vi "Main.vi"(11 "Module Admin":refnum<class "Delacor_lib_QMH_Module Admin.lvclass">) -> ()   [LabVIEW 2022 SP3, in "UI Manager.lvlib"]
doc: "The UI Manager module forms the visual framework that other modules are displayed in. It contains the basic user interface of the application (menu bar, header, content area, footer).\n____\nHAMPEL SOFTWARE ENGINEERING v2.6.0 (2023-12-19 10:54)"
uses:
  UI Manager.lvlib
  <vilib>/Delacor/Delacor QMH/Libraries/Module Admin_class/Delacor_lib_QMH_Module Admin.lvclass
  Libraries/hse-libraries/Source/hse-dqmh/Controls/System Message Argument--cluster.ctl
  Libraries/hse-libraries/Source/hse-dqmh/Controls/System Message Source.ctl
  Module Data--cluster.ctl
  Libraries/hse-libraries/Source/hse-configuration/config-base/config-base.lvclass
  SubVIs/Layout References--cluster.ctl
  SubVIs/SubPanels--map.ctl
  SubVIs/SubPnl Map References--cluster.ctl
  Login Argument--cluster.ctl
  <vilib>/Delacor/Delacor QMH/Libraries/Message Queue_class/Delacor_lib_QMH_Message Queue.lvclass/Delacor_lib_QMH_Message Queue.ctl
  Stop Argument--cluster.ctl
  Shutdown Application Argument--cluster.ctl
  Add Module to Run-Time Menu Argument--cluster.ctl
  Libraries/hse-libraries/Source/hse-dqmh/Controls/System Message - Add to Run-Time Menu - Argument--cluster.ctl
  Remove Module from Run-Time Menu Argument--cluster.ctl
  Libraries/hse-libraries/Source/hse-dqmh/Controls/System Message - Remove from Run-Time Menu - Argument--cluster.ctl
  Load Module Into Subpanel Argument--cluster.ctl
  Libraries/hse-libraries/Source/hse-dqmh/Controls/System Message - Ready for Display - Payload--cluster.ctl
  Configure Argument--cluster.ctl
  Prepare Argument--cluster.ctl
  Set Modules Argument--cluster.ctl
  Set Modules (Reply Payload)--cluster.ctl
  Set Run-Time Menu Argument--cluster.ctl
  Show HSE-ABOUT Argument--cluster.ctl
  Show PROJECT-ABOUT Argument--cluster.ctl
  Update Status Bar Argument--cluster.ctl
  Trigger System Message Argument--cluster.ctl
  Display another Module UI Argument--cluster.ctl
  Module Display Scenarios.ctl
  Set Run-Time Menu Visibility Argument--cluster.ctl
  Set Window Closeable State Argument--cluster.ctl
  Set CLI Arguments Argument--cluster.ctl
  Set CLI Arguments (Reply Payload)--cluster.ctl
  Get CLI Arguments Argument--cluster.ctl
  Get CLI Arguments (Reply Payload)--cluster.ctl
  External Login Argument--cluster.ctl
  Get User Level Argument--cluster.ctl
  Get User Level (Reply Payload)--cluster.ctl
  <vilib>/Delacor/Delacor QMH/Libraries/Module Admin_class/Delacor_lib_QMH_Module Admin.lvclass/Delacor_lib_QMH_Module Admin.ctl
  Libraries/hse-libraries/Source/hse-application/hse-application.lvclass/hse-application.ctl
  <vilib>/Delacor/Delacor QMH/Libraries/Message Queue_class/Delacor_lib_QMH_Enqueue Message (Single).vi
  <vilib>/Delacor/Delacor QMH/Libraries/Module Admin_class/Delacor_lib_QMH_Get External Launch.vi
  Libraries/hse-libraries/Source/hse-application/HSE Application not initialized--error.vi
  Libraries/hse-libraries/Source/hse-configuration/config-ini/config-ini.lvclass
  C:/Projects/579-Intelligent-Systems-Term-Project/06_Source/UI/FReVSys_Source/Libraries/hse-libraries/Source/hse-configuration/config-base/config-base.lvclass
  Libraries/hse-libraries/Source/hse-application/hse-application__GetSingleton.vi
  <vilib>/Utility/error.llb/Error Cluster From Error Code.vi
  Project/PROJECT_Evaluate Default Menu Selection.vi
  Project/PROJECT_UserCredentials.vi
  <vilib>/ErrorRing/Error Ring.xnode
  <vilib>/Delacor/Delacor QMH/Libraries/Message Queue_class/Delacor_lib_QMH_Message Queue.lvclass
  Libraries/hse-libraries/Source/hse-ui/hse-ui.lvlib
  Libraries/hse-libraries/Source/hse-application/hse-application.lvclass
  Libraries/hse-libraries/Source/hse-dqmh/hse-dqmh.lvlib
  <vilib>/Hampel Software Engineering/HSE Logger/hse-logger.lvlib
  Project/Project.lvlib
panel:
  out "Status Bar":string
  out "error out":errorcluster
  out "Version":string
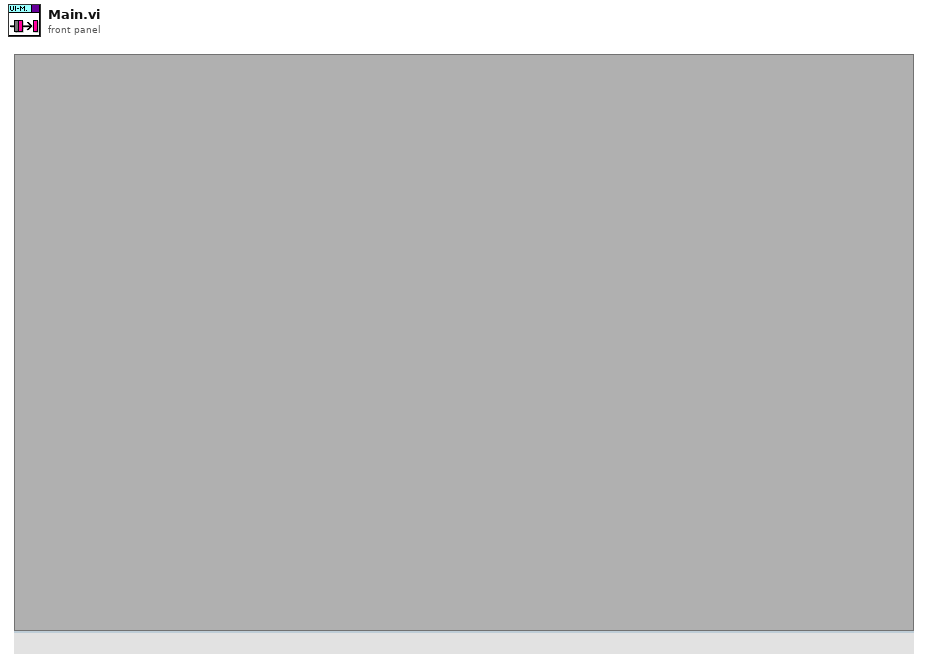
[diagram p1: front panel]
types:
  T1 = typedef "UI Manager.lvlib/Request Events--cluster.ctl" = cluster{"Stop Module":refnum<user-event>, "Show Panel":refnum<user-event>, "Hide Panel":refnum<user-event>, "Get Module Execution Status":refnum<user-event>, "Show Diagram":refnum<user-event>, "Set Run-Time Menu":refnum<user-event>, "Show HSE-ABOUT":refnum<user-event>, "Show PROJECT-ABOUT":refnum<user-event>, "Configure":refnum<user-event>, "Prepare":refnum<user-event>, "Update Status Bar":refnum<user-event>, "Trigger System Message":refnum<user-event>, "Add Module to Run-Time Menu":refnum<user-event>, "Set Modules":refnum<user-event>, "Register for Module Events":refnum<user-event>, "Display another Module UI":refnum<user-event>, "Set Run-Time Menu Visibility":refnum<user-event>, "Set Window Closeable State":refnum<user-event>, "Shutdown Application":refnum<user-event>, "Remove Module from Run-Time Menu":refnum<user-event>, "Set CLI Arguments":refnum<user-event>, "Get CLI Arguments":refnum<user-event>, "External Login":refnum<user-event>, "Get User Level":refnum<user-event>}
  T2 = typedef "UI Manager.lvlib/Module Data--cluster.ctl" = cluster{"hse-config":refnum<class "config-base.lvclass">, "Module Paths":path[], "Default Title":string, "Layout":T3, "CLI Arguments":string[], "Login Argument":T6}
  T3 = typedef "UI Manager.lvlib/Layout References--cluster.ctl" = cluster{"Layout-VI Ref":refnum<vi>, "SP_Content Ref":refnum<vi>, "Subpanel VI Ref":refnum<vi>, "STR_Headline":refnum<vi>, "SubPanels":T4}
  T4 = typedef "UI Manager.lvlib/SubPanels--map.ctl" = map{string, T5}
  T5 = typedef "UI Manager.lvlib/SubPnl Map References--cluster.ctl" = cluster{"SubPnl Refnum":refnum<vi>, "VI Refnum":refnum<vi>}
  T6 = typedef "UI Manager.lvlib/Login Argument--cluster.ctl" = cluster{"User Name":string, "User Level":string}
  T7 = enum32{"invalid lock state", "Not Locked", "Locked (No Password)", "Password-protected"}
  T8 = typedef "UI Manager.lvlib/Stop Argument--cluster.ctl" = cluster{"Origin":string, "Exit via Stop Module Req?":bool, "Wait for Module to stop?":bool}
  T9 = typedef "UI Manager.lvlib/Shutdown Application Argument--cluster.ctl" = cluster{"User Confirm?":bool}
  T10 = typedef "hse-dqmh.lvlib/System Message - Add to Run-Time Menu - Argument--cluster.ctl" = cluster{"Module Disk Path":path, "Module Descriptor":string}
  T11 = typedef "UI Manager.lvlib/Add Module to Run-Time Menu Argument--cluster.ctl" = cluster{"Module DQMH Path":path, "Module Descriptor":string}
  T12 = typedef "hse-dqmh.lvlib/System Message - Remove from Run-Time Menu - Argument--cluster.ctl" = cluster{"Module Disk Path":path}
  T13 = typedef "UI Manager.lvlib/Remove Module from Run-Time Menu Argument--cluster.ctl" = cluster{"Module DQMH Path":path}
  T14 = typedef "hse-dqmh.lvlib/System Message - Ready for Display - Payload--cluster.ctl" = cluster{"Module Path":path, "VI Reference":refnum<vi>, "Title":string, "Target SP Name":string}
  T15 = typedef "UI Manager.lvlib/Load Module Into Subpanel Argument--cluster.ctl" = cluster{"Module Path":path, "Module Name":string, "Title":string, "VI Reference":refnum<vi>, "Target SP Name":string}
  T16 = typedef "UI Manager.lvlib/Configure Argument--cluster.ctl" = cluster{"Boolean":bool}
  T17 = typedef "UI Manager.lvlib/Prepare Argument--cluster.ctl" = cluster{"Boolean":bool}
  T18 = typedef "UI Manager.lvlib/Set Modules Argument--cluster.ctl" = cluster{"Module Paths":path[], "Wait Notifier":refnum<notifier>, "wait for reply":bool}
  T19 = typedef "UI Manager.lvlib/Set Run-Time Menu Argument--cluster.ctl" = cluster{"Run-Time Menu Path":path}
  T20 = typedef "UI Manager.lvlib/Show HSE-ABOUT Argument--cluster.ctl" = cluster{"Boolean":bool}
  T21 = typedef "UI Manager.lvlib/Show PROJECT-ABOUT Argument--cluster.ctl" = cluster{"Boolean":bool}
  T22 = typedef "UI Manager.lvlib/Update Status Bar Argument--cluster.ctl" = cluster{"Status Message":string}
  T23 = typedef "UI Manager.lvlib/Trigger System Message Argument--cluster.ctl" = cluster{"Boolean":bool}
  T24 = typedef "UI Manager.lvlib/Display another Module UI Argument--cluster.ctl" = cluster{"Module DQMH Path":path, "Display Scenario":T25}
  T25 = typedef "UI Manager.lvlib/Module Display Scenarios.ctl" = enum16{"Stand-Alone", "Managed"}
  T26 = typedef "UI Manager.lvlib/Set Run-Time Menu Visibility Argument--cluster.ctl" = cluster{"Visible?":bool}
  T27 = typedef "UI Manager.lvlib/Set Window Closeable State Argument--cluster.ctl" = cluster{"Closeable?":bool}
  T28 = typedef "UI Manager.lvlib/Set CLI Arguments Argument--cluster.ctl" = cluster{"CLI Arguments":string[], "Wait Notifier":refnum<notifier>, "wait for reply":bool}
  T29 = typedef "UI Manager.lvlib/Get CLI Arguments Argument--cluster.ctl" = cluster{"Wait Notifier":refnum<notifier>, "wait for reply":bool}
  T30 = typedef "UI Manager.lvlib/External Login Argument--cluster.ctl" = cluster{"User Name":string, "User Level":string}
  T31 = typedef "UI Manager.lvlib/Get User Level Argument--cluster.ctl" = cluster{"Wait Notifier":refnum<notifier>, "wait for reply":bool}
  T32 = enum32{"Invalid", "Standard", "Closed", "Hidden", "Minimized", "Maximized"}
  T33 = typedef "UI Manager.lvlib/Set Modules (Reply Payload)--cluster.ctl" = cluster{"error":errorcluster}
  T34 = typedef "UI Manager.lvlib/Set CLI Arguments (Reply Payload)--cluster.ctl" = cluster{"error":errorcluster}
  T35 = typedef "UI Manager.lvlib/Get CLI Arguments (Reply Payload)--cluster.ctl" = cluster{"CLI Arguments":string[], "error":errorcluster}
  T36 = typedef "UI Manager.lvlib/Get User Level (Reply Payload)--cluster.ctl" = cluster{"User Name":string, "User Level":string, "error":errorcluster}
  T37 = typedef "eventvkey.ctl" = enum16{"ASCII", "Enter", "Return", "Shift", "Ctrl", "Alt", "Cmd", "Opt", "Caps", "NumLock", "Clear", "Break", "Up", "Down", "Left", "Right", "Insert", "Delete", "Home", "End", "PageUp", "PageDown", "Escape", "Help", "Pause", "ScrollLock", "F1", "F2", "F3", "F4", "F5", "F6", "F7", "F8", "F9", "F10", "F11", "F12", "F13", "F14", "F15", "F16", "F17", "F18", "F19", "F20", "F21", "F22", "F23", "F24", "Play", "VolumeUp", "VolumeDown", "Mute", "Two Byte Char"}
  T38 = cluster{"Shift":bool, "Ctrl":bool, "Alt":bool, "Cmd":bool, "Opt":bool}
  T39 = typedef "hse-dqmh.lvlib/System Message Source.ctl" = enum16{"module", "application", "network"}
  T40 = typedef "hse-dqmh.lvlib/Module Types.ctl" = enum16{"Singleton", "Cloneable"}
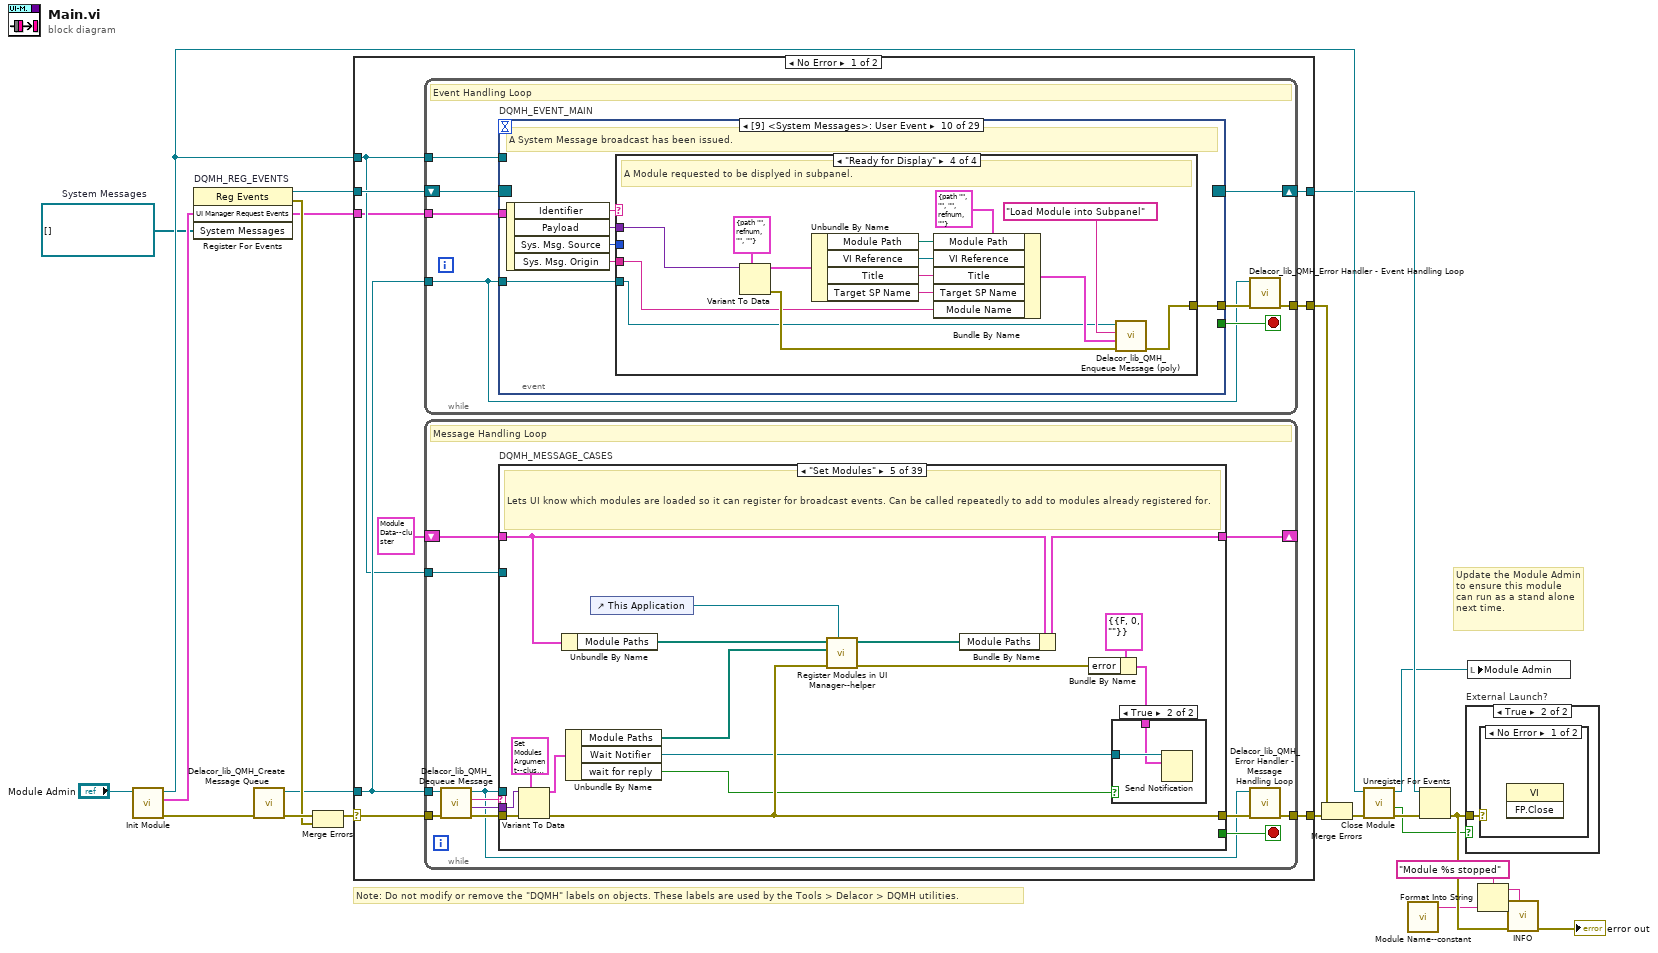
[diagram p0: block diagram]
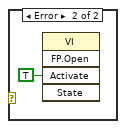
[diagram p3: hidden frame]
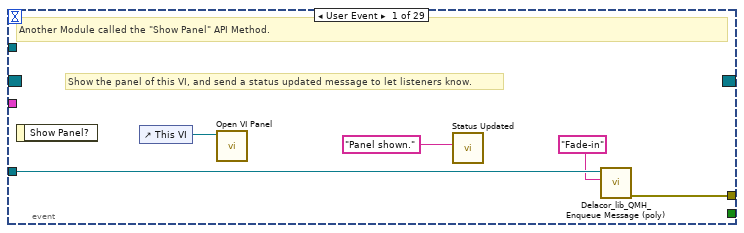
[diagram p4: hidden frame]
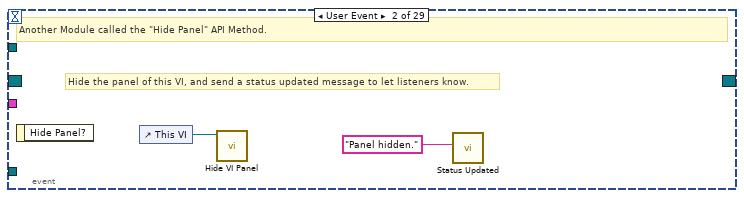
[diagram p5: hidden frame]
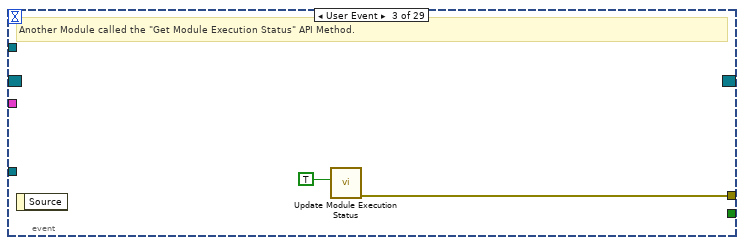
[diagram p6: hidden frame]
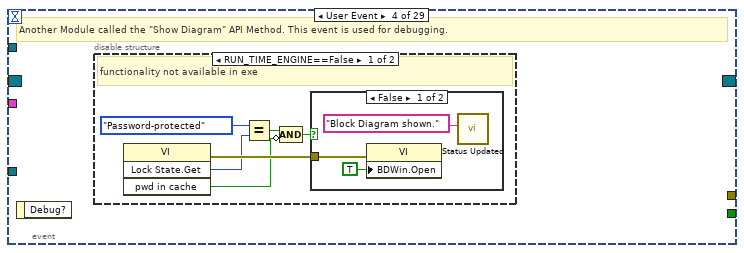
[diagram p7: hidden frame]
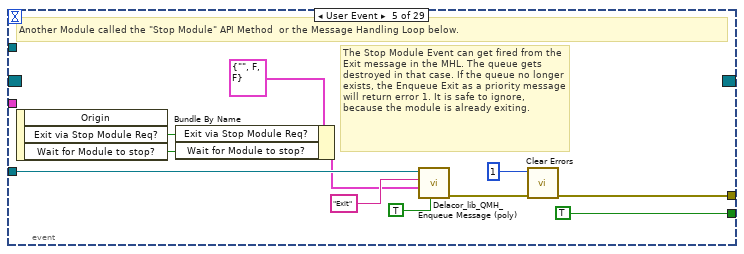
[diagram p10: hidden frame]
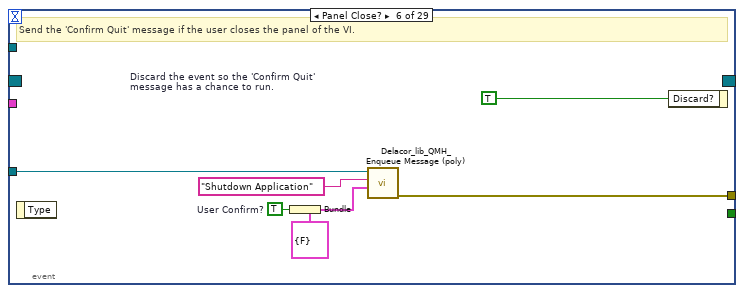
[diagram p11: hidden frame]
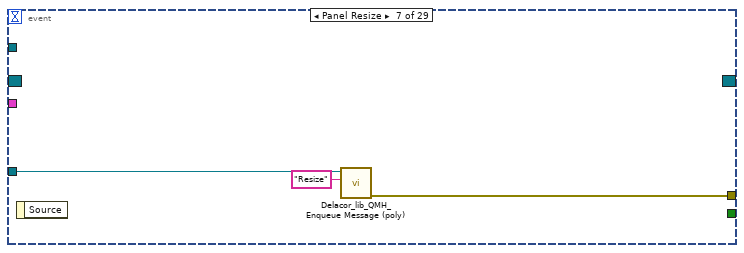
[diagram p12: hidden frame]
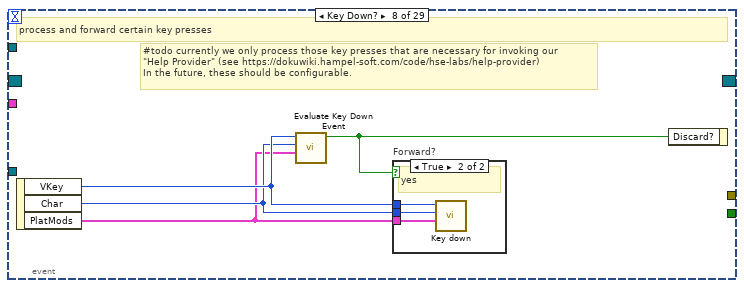
[diagram p13: hidden frame]
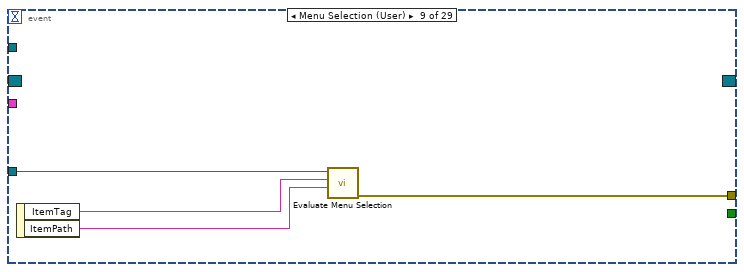
[diagram p15: hidden frame]
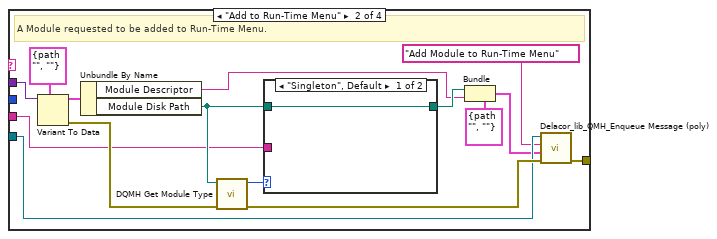
[diagram p17: hidden frame]
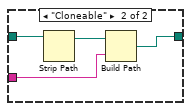
[diagram p18: hidden frame]
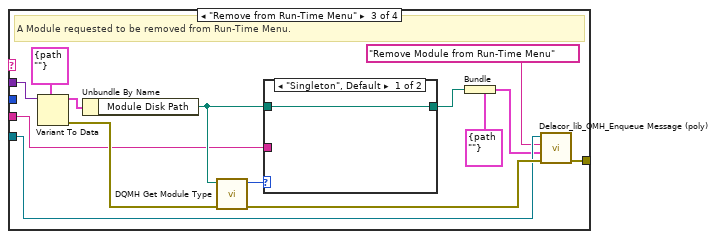
[diagram p19: hidden frame]
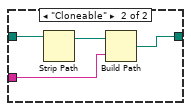
[diagram p20: hidden frame]
diagram:
  w5 = refnum<user-event>[] []  # System Messages
  # "Note: Do not modify or remove the \"DQMH\" labels on objects. These labels are used by the Tools > Delacor > DQMH utilities."
  # "Update the Module Admin to ensure this module can run as a stand alone next time."
  n1 = call "Init Module.vi"("Singleton Module Admin in"="Module Admin") -> ("error out"=w21:errorcluster, "UI Manager Request Events"=w6:T1, "Singleton Module Admin out"=w12:refnum<class "Delacor_lib_QMH_Module Admin.lvclass">)  [unwired: 8 in]
  n2 = register-events "DQMH_REG_EVENTS"(w6, w5) -> (reference out=w10:refnum<event-registration>, error out=w15:errorcluster)  [unwired: 2 in]
  n3 = call <vilib>:"Delacor_lib_QMH_Create Message Queue.vi"("error in"=w21) -> ("error out"=w17:errorcluster, "Message Queue"=w9:refnum<class "Delacor_lib_QMH_Message Queue.lvclass">)  [unwired: 9 in]
  n4 = Merge Errors(w17, w15) -> (w16:errorcluster)
  n5 = case shown="No Error" w16 {
    selector: w16 -> [w29 w779]
    tunnel: [w31 w779] -> w22
    tunnel: [w28 w776] -> w11
    tunnel: w10 -> [w26 w776]
    tunnel: w9 -> [w25 w771]
    tunnel: [w30 _] -> w19
    tunnel: w12 -> [w24 w772]
    tunnel: w6 -> [w23 _]
    frame No Error {
      n6 = while {
        tunnel: w25 -> [w34]
        shift-right: [w37] -> w28
        shift-left: w26 -> [w32]
        tunnel: [w38] -> w30
        tunnel: w24 -> [w35]
        tunnel: w23 -> [w33]
        stop <- w36 stop-if-true
        # "Event Handling Loop"
        n7 = event "DQMH_EVENT_MAIN" shown="[9] <System Messages>: User Event" {
          selector: w32 -> [_ _ _ _ _ _ _ _ _ _ _ _ _ w171 _ _ _ _ _ _ _ _ _ _ _ _ _ _ _]
          dyn-events: [_ _ _ _ _ _ _ _ _ _ _ _ _ w170 _ _ _ _ _ _ _ _ _ _ _ _ _ _ _] -> w37
          timeout: _ -> [_ _ _ _ _ _ _ _ _ _ _ _ _ _ _ _ _ _ _ _ _ _ _ _ _ _ _ _ _]
          tunnel: [_ _ _ _ TRUE ("Discard?") _ _ _ _ _ _ _ _ _ _ _ _ _ _ _ _ _ _ _ _ _ _ _ _] -> w36
          tunnel: w34 -> [w41 _ _ _ w64 w73 w76 _ w88 w94 w153 w159 w167 _ w177 w184 w190 w196 w202 w208 w215 w221 w227 w233 w239 w247 w255 w259 w266]
          tunnel: [w42 _ w48 _ w67 w75 w78 _ w89 w95 w154 w160 w168 w172 w178 w185 w191 w197 w203 w209 w216 w222 w228 w234 w240 w248 w249 w258 w265] -> w39
          tunnel: w35 -> [_ _ _ _ _ _ _ _ _ _ _ _ _ _ _ _ _ _ _ _ _ _ _ _ _ _ _ _ _]
          tunnel: w33 -> [_ _ _ _ _ _ _ _ _ _ _ _ _ _ _ _ _ _ _ _ _ _ _ _ _ _ _ _ _]
          event User Event {
            # "Show the panel of this VI, and send a status updated message to let listeners know."
            # "Another Module called the \"Show Panel\" API Method."
            n8 = event-data() -> ()  [unwired: 1 in, 1 out]
            n9 = control-ref of="This VI"() -> (w44:refnum<vi>)
            n10 = call "Open VI Panel.vi"("VI"=w44) -> ()  [unwired: 10 in, 1 out]
            n11 = call "Status Updated.vi"("Status"="Panel shown." ("format string")) -> ()  [unwired: 10 in, 1 out]
            n12 = call-poly <vilib>:"Delacor_lib_QMH_Enqueue Message (poly).vi"("Message"="Fade-in", "Message Queue in"=w41) -> ("error out"=w42:errorcluster)  [unwired: 8 in, 1 out]
          }
          event User Event {
            # "Hide the panel of this VI, and send a status updated message to let listeners know."
            # "Another Module called the \"Hide Panel\" API Method."
            n13 = event-data() -> ()  [unwired: 1 in, 1 out]
            n14 = control-ref of="This VI"() -> (w46:refnum<vi>)
            n15 = call "Hide VI Panel.vi"("VI"=w46) -> ()  [unwired: 10 in, 1 out]
            n16 = call "Status Updated.vi"("Status"="Panel hidden." ("format string")) -> ()  [unwired: 10 in, 1 out]
          }
          event User Event {
            # "Another Module called the \"Get Module Execution Status\" API Method."
            n17 = event-data() -> ()  [unwired: 1 in, 1 out]
            n18 = call "Update Module Execution Status.vi"("Running?"=TRUE) -> ("error out"=w48:errorcluster)  [unwired: 10 in]
          }
          event User Event {
            # "Another Module called the \"Show Diagram\" API Method. This event is used for debugging."
            n19 = event-data() -> ()  [unwired: 1 in, 1 out]
            n20 = disable-structure shown="RUN_TIME_ENGINE==False" {
              frame condition #0 (active) {
                # "functionality not available in exe"
                n21 = invoke on="Invoke Node" class="VI" method="Lock State.Get"() -> (error out=w54:errorcluster, "Get Lock State"=w53:T7, "pwd in cache"=w50:bool)  [unwired: 4 in, 1 out]
                n22 = Equal?(x=T7."Password-protected", y=w53) -> (x = y?=w51:bool)
                n23 = Compound Arithmetic op=AND(w51, invert w50) -> (w49:bool)
                n24 = case shown="False" w49 {
                  tunnel: w54 -> [w57 _]
                  frame False {
                    n25 = property on="Property Node" class="VI"(error in=w57, "BDWin.Open"=TRUE ("Block Diagram Window:Open")) -> ()  [unwired: 1 in, 2 out]
                    n26 = call "Status Updated.vi"("Status"="Block Diagram shown." ("format string")) -> ()  [unwired: 10 in, 1 out]
                  }
                  frame True {
                    # "Password-protected VI, and the password is not in the cache. Do not show the diagram."
                  }
                }
              }
              frame condition #1 {
              }
            }
          }
          event User Event {
            # "The Stop Module Event can get fired from the Exit message in the MHL. The queue gets destroyed in that case. If the queue no longer exists, the Enqueue Exit as a priority message will return error 1. It is safe to ignore, because the module is already exiting."
            # "Another Module called the \"Stop Module\" API Method  or the Message Handling Loop below."
            n27 = event-data() -> ("Exit via Stop Module Req?"=w60:bool, "Wait for Module to stop?"=w59:bool)  [unwired: 1 in, 1 out]
            n28 = Bundle By Name(cluster=T8 {"Origin"="", "Exit via Stop Module Req?"=FALSE, "Wait for Module to stop?"=FALSE} ("Stop Argument"), "Exit via Stop Module Req?"=w60, "Wait for Module to stop?"=w59) -> (w58:T8)
            n29 = call-poly <vilib>:"Delacor_lib_QMH_Enqueue Message (poly).vi"("Priority Message? (F)"=TRUE, "Message Data"=w58, "Message"="Exit", "Message Queue in"=w64) -> ("error out"=w68:errorcluster)  [unwired: 6 in, 1 out]
            n30 = call <vilib>:"Clear Errors.vi"("error in (no error)"=w68, "specific error code to clear (0: all)"=1) -> ("error out"=w67:errorcluster)  [unwired: 4 in, 1 out]
          }
          event Panel Close? {
            w69 = TRUE  # User Confirm?
            w74 = TRUE  # Discard the event so the 'Confirm Quit' message has a chance to run.
            # "Send the 'Confirm Quit' message if the user closes the panel of the VI."
            n31 = event-data() -> ()  [unwired: 1 in, 1 out]
            n32 = Bundle(cluster=T9 {"User Confirm?"=FALSE} ("Shutdown Application Argument"), "User Confirm?"=w69) -> (w70:T9)
            n33 = call-poly <vilib>:"Delacor_lib_QMH_Enqueue Message (poly).vi"("Message Data"=w70, "Message"="Shutdown Application", "Message Queue in"=w73) -> ("error out"=w75:errorcluster)  [unwired: 7 in, 1 out]
            n34 = event-data ("Event Filter Node")("Discard?"=w74) -> ()  [unwired: 1 in, 1 out]
          }
          event Panel Resize {
            n35 = event-data() -> ()  [unwired: 1 in, 1 out]
            n36 = call-poly <vilib>:"Delacor_lib_QMH_Enqueue Message (poly).vi"("Message"="Resize", "Message Queue in"=w76) -> ("error out"=w78:errorcluster)  [unwired: 8 in, 1 out]
          }
          event Key Down? {
            # "#todo currently we only process those key presses that are necessary for invoking our \n\"Help Provider\" (see https://dokuwiki.hampel-soft.com/code/hse-labs/help-provider)\nIn the future, these should be configurable."
            # "process and forward certain key presses"
            n37 = event-data() -> ("VKey"=w82:T37, "Char"=w81:i16, "PlatMods"=w80:T38)  [unwired: 1 in]
            n38 = call "Evaluate Key Down Event.vi"("PlatMods"=w80, "Char"=w81, "VKey"=w82) -> ("do forward"=w79:bool)  [unwired: 8 in]
            n39 = case "Forward?" shown="True" w79 {
              tunnel: w82 -> [_ w85]
              tunnel: w81 -> [_ w84]
              tunnel: w80 -> [_ w83]
              frame False {
                # "no"
              }
              frame True {
                # "yes"
                n40 = call "Key down.vi"("PlatMods"=w83, "Char"=w84, "VKey"=w85) -> ()  [unwired: 8 in, 1 out]
              }
            }
            n41 = event-data ("Event Filter Node")("Discard?"=w79) -> ()  [unwired: 1 in, 1 out]
          }
          event Menu Selection (User) {
            n42 = event-data() -> ("ItemTag"=w87:string, "ItemPath"=w86:string)  [unwired: 1 in]
            n43 = call "Evaluate Menu Selection.vi"("ItemPath"=w86, "ItemTag"=w87, "MQ in"=w88) -> ("error out"=w89:errorcluster)  [unwired: 8 in]
          }
          event User Event {
            # "A System Message broadcast has been issued."
            n44 = event-data() -> ("Identifier"=w93:string, "Payload"=w92:variant, "Sys. Msg. Source"=w91:T39, "Sys. Msg. Origin"=w90:string)  [unwired: 1 in]
            n45 = case shown="\"Ready for Display\"" w93 {
              tunnel: w94 -> [_ w107 w126 w137]
              tunnel: [_ w109 w128 w148] -> w95
              tunnel: w92 -> [_ w103 w123 w145]
              tunnel: w91 -> [_ _ _ _]
              tunnel: w90 -> [_ w97 w118 w136]
              frame Default {
              }
              frame "Add to Run-Time Menu" {
                # "A Module requested to be added to Run-Time Menu."
                n46 = Variant To Data(type=T10 {"Module Disk Path"=path "", "Module Descriptor"=""} ("Add to RTM Argument"), Variant=w103) -> (data=w101:T10, error out=w108:errorcluster)  [unwired: 1 in]
                n47 = Unbundle By Name(w101) -> ("Module Descriptor"=w96:string, "Module Disk Path"=w99:path)
                n48 = call "DQMH Get Module Type.vi"("error in"=w108, "Module Path"=w99) -> ("error out"=w110:errorcluster, "Module Types"=w100:T40)  [unwired: 8 in]
                n49 = case shown="\"Singleton\", Default" w100 {
                  tunnel: [w111 w112] -> w98
                  tunnel: w99 -> [w111 w114]
                  tunnel: w97 -> [_ w113]
                  frame "Singleton", Default {
                  }
                  frame "Cloneable" {
                    n50 = Strip Path(path=w114) -> (stripped path=w115:path)  [unwired: 1 out]
                    n51 = Build Path(base path=w115, name or relative path=w113) -> (appended path=w112:path)
                  }
                }
                n52 = Bundle(cluster=T11 {"Module DQMH Path"=path "", "Module Descriptor"=""} ("Add Module to Run-Time Menu Argument"), "Module DQMH Path"=w98, "Module Descriptor"=w96) -> (w104:T11)
                n53 = call-poly <vilib>:"Delacor_lib_QMH_Enqueue Message (poly).vi"("error in"=w110, "Message Data"=w104, "Message"="Add Module to Run-Time Menu", "Message Queue in"=w107) -> ("error out"=w109:errorcluster)  [unwired: 6 in, 1 out]
              }
              frame "Remove from Run-Time Menu" {
                # "A Module requested to be removed from Run-Time Menu."
                n54 = Variant To Data(type=T12 {"Module Disk Path"=path ""} ("Remove fromRTM Argument"), Variant=w123) -> (data=w122:T12, error out=w127:errorcluster)  [unwired: 1 in]
                n55 = Unbundle By Name(w122) -> ("Module Disk Path"=w120:path)
                n56 = call "DQMH Get Module Type.vi"("error in"=w127, "Module Path"=w120) -> ("error out"=w129:errorcluster, "Module Types"=w121:T40)  [unwired: 8 in]
                n57 = case shown="\"Singleton\", Default" w121 {
                  tunnel: [w130 w131] -> w119
                  tunnel: w120 -> [w130 w133]
                  tunnel: w118 -> [_ w132]
                  frame "Singleton", Default {
                  }
                  frame "Cloneable" {
                    n58 = Strip Path(path=w133) -> (stripped path=w134:path)  [unwired: 1 out]
                    n59 = Build Path(base path=w134, name or relative path=w132) -> (appended path=w131:path)
                  }
                }
                n60 = Bundle(cluster=T13 {"Module DQMH Path"=path ""} ("Remove Module from Run-Time Menu Argument"), "Module DQMH Path"=w119) -> (w124:T13)
                n61 = call-poly <vilib>:"Delacor_lib_QMH_Enqueue Message (poly).vi"("error in"=w129, "Message Data"=w124, "Message"="Remove Module from Run-Time Menu", "Message Queue in"=w126) -> ("error out"=w128:errorcluster)  [unwired: 6 in, 1 out]
              }
              frame "Ready for Display" {
                # "A Module requested to be displyed in subpanel."
                n62 = Variant To Data(type=T14 {"Module Path"=path "", "VI Reference"=refnum, "Title"="", "Target SP Name"=""} ("Ready for Display Payload"), Variant=w145) -> (data=w141:T14, error out=w147:errorcluster)  [unwired: 1 in]
                n63 = Unbundle By Name(w141) -> ("Module Path"=w140:path, "VI Reference"=w139:refnum<vi>, "Title"=w138:string, "Target SP Name"=w135:string)
                n64 = Bundle By Name(cluster=T15 {"Module Path"=path "", "Module Name"="", "Title"="", "VI Reference"=refnum, "Target SP Name"=""} ("Load Module Into Subpanel Argument"), "Module Path"=w140, "VI Reference"=w139, "Title"=w138, "Target SP Name"=w135, "Module Name"=w136) -> (w144:T15)
                n65 = call-poly <vilib>:"Delacor_lib_QMH_Enqueue Message (poly).vi"("error in"=w147, "Message Data"=w144, "Message"="Load Module into Subpanel", "Message Queue in"=w137) -> ("error out"=w148:errorcluster)  [unwired: 6 in, 1 out]
              }
            }
          }
          event User Event {
            # "Another Module called the \"Configure\" API Method."
            n66 = event-data() -> ("Boolean"=w149:bool)  [unwired: 1 in]
            n67 = Bundle(cluster=T16 {"Boolean"=FALSE} ("Configure Argument"), "Boolean"=w149) -> (w150:T16)
            n68 = call-poly <vilib>:"Delacor_lib_QMH_Enqueue Message (poly).vi"("Message Data"=w150, "Message"="Configure", "Message Queue in"=w153) -> ("error out"=w154:errorcluster)  [unwired: 7 in, 1 out]
          }
          event User Event {
            # "Another Module called the \"Prepare\" API Method."
            n69 = event-data() -> ("Boolean"=w155:bool)  [unwired: 1 in]
            n70 = Bundle(cluster=T17 {"Boolean"=FALSE} ("Prepare Argument"), "Boolean"=w155) -> (w156:T17)
            n71 = call-poly <vilib>:"Delacor_lib_QMH_Enqueue Message (poly).vi"("Message Data"=w156, "Message"="Prepare", "Message Queue in"=w159) -> ("error out"=w160:errorcluster)  [unwired: 7 in, 1 out]
          }
          event User Event {
            # "Another Module called the \"Set Modules\" API Method."
            n72 = event-data() -> ("Module Paths"=w163:path[], "Wait Notifier"=w162:refnum<notifier>, "wait for reply"=w161:bool)  [unwired: 1 in]
            n73 = Bundle(cluster=T18 {"Module Paths"=[path "Modules/Dummie"], "Wait Notifier"=refnum, "wait for reply"=FALSE} ("Set Modules Argument"), "Module Paths"=w163, "Wait Notifier"=w162, "wait for reply"=w161) -> (w164:T18)
            n74 = call-poly <vilib>:"Delacor_lib_QMH_Enqueue Message (poly).vi"("Message Data"=w164, "Message"="Set Modules", "Message Queue in"=w167) -> ("error out"=w168:errorcluster)  [unwired: 7 in, 1 out]
          }
          event User Event {
            # "The MHL called the private \"Register for Module Events\" API Method."
            n75 = event-data() -> ("System Messages"=w169:refnum<user-event>[])  [unwired: 1 in]
            n76 = register-events "DQMH_REG_EVENTS_INSIDE_LOOP"(reference=w171, w169) -> (reference out=w170:refnum<event-registration>, error out=w172:errorcluster)  [unwired: 2 in]
          }
          event User Event {
            # "Another Module called the \"Set Run-Time Menu\" API Method."
            n77 = event-data() -> ("Run-Time Menu Path"=w173:path)  [unwired: 1 in]
            n78 = Bundle(cluster=T19 {"Run-Time Menu Path"=path ""} ("Set Run-Time Menu Argument"), "Run-Time Menu Path"=w173) -> (w174:T19)
            n79 = call-poly <vilib>:"Delacor_lib_QMH_Enqueue Message (poly).vi"("Message Data"=w174, "Message"="Set Run-Time Menu", "Message Queue in"=w177) -> ("error out"=w178:errorcluster)  [unwired: 7 in, 1 out]
          }
          event User Event {
            # "Another Module called the \"Add Module to Run-Time Menu\" API Method."
            n80 = event-data() -> ("Module DQMH Path"=w180:path, "Module Descriptor"=w179:string)  [unwired: 1 in]
            n81 = Bundle(cluster=T11 {"Module DQMH Path"=path "", "Module Descriptor"=""} ("Add Module to Run-Time Menu Argument"), "Module DQMH Path"=w180, "Module Descriptor"=w179) -> (w181:T11)
            n82 = call-poly <vilib>:"Delacor_lib_QMH_Enqueue Message (poly).vi"("Message Data"=w181, "Message"="Add Module to Run-Time Menu", "Message Queue in"=w184) -> ("error out"=w185:errorcluster)  [unwired: 7 in, 1 out]
          }
          event User Event {
            # "Another Module called the \"Show HSE-ABOUT\" API Method."
            n83 = event-data() -> ("Boolean"=w186:bool)  [unwired: 1 in]
            n84 = Bundle(cluster=T20 {"Boolean"=FALSE} ("Show HSE-ABOUT Argument"), "Boolean"=w186) -> (w187:T20)
            n85 = call-poly <vilib>:"Delacor_lib_QMH_Enqueue Message (poly).vi"("Message Data"=w187, "Message"="Show HSE-ABOUT", "Message Queue in"=w190) -> ("error out"=w191:errorcluster)  [unwired: 7 in, 1 out]
          }
          event User Event {
            # "Another Module called the \"Show PROJECT-ABOUT\" API Method."
            n86 = event-data() -> ("Boolean"=w192:bool)  [unwired: 1 in]
            n87 = Bundle(cluster=T21 {"Boolean"=FALSE} ("Show PROJECT-ABOUT Argument"), "Boolean"=w192) -> (w193:T21)
            n88 = call-poly <vilib>:"Delacor_lib_QMH_Enqueue Message (poly).vi"("Message Data"=w193, "Message"="Show PROJECT-ABOUT", "Message Queue in"=w196) -> ("error out"=w197:errorcluster)  [unwired: 7 in, 1 out]
          }
          event User Event {
            # "Another Module called the \"Update Status Bar\" API Method."
            n89 = event-data() -> ("Status Message"=w198:string)  [unwired: 1 in]
            n90 = Bundle(cluster=T22 {"Status Message"=""} ("Update Status Bar Argument"), "Status Message"=w198) -> (w199:T22)
            n91 = call-poly <vilib>:"Delacor_lib_QMH_Enqueue Message (poly).vi"("Message Data"=w199, "Message"="Update Status Bar", "Message Queue in"=w202) -> ("error out"=w203:errorcluster)  [unwired: 7 in, 1 out]
          }
          event User Event {
            # "Another Module called the \"Trigger System Message\" API Method."
            n92 = event-data() -> ("Boolean"=w205:bool)  [unwired: 1 in]
            n93 = Bundle(cluster=T23 {"Boolean"=FALSE} ("Trigger System Message Argument"), "Boolean"=w205) -> (w206:T23)
            n94 = call-poly <vilib>:"Delacor_lib_QMH_Enqueue Message (poly).vi"("Message Data"=w206, "Message"="Trigger System Message", "Message Queue in"=w208) -> ("error out"=w209:errorcluster)  [unwired: 7 in, 1 out]
          }
          event User Event {
            # "Another Module called the \"Display Module UI\" API Method."
            n95 = event-data() -> ("Module DQMH Path"=w211:path, "Display Scenario"=w210:T25)  [unwired: 1 in]
            n96 = Bundle(cluster=T24 {"Module DQMH Path"=path "", "Display Scenario"=enum."Stand-Alone"} ("Display Module UI Argument"), "Module DQMH Path"=w211, "Display Scenario"=w210) -> (w212:T24)
            n97 = call-poly <vilib>:"Delacor_lib_QMH_Enqueue Message (poly).vi"("Message Data"=w212, "Message"="Display another Module UI", "Message Queue in"=w215) -> ("error out"=w216:errorcluster)  [unwired: 7 in, 1 out]
          }
          event User Event {
            # "Another Module called the \"Set Run-Time Menu Visibility\" API Method."
            n98 = event-data() -> ("Visible?"=w217:bool)  [unwired: 1 in]
            n99 = Bundle(cluster=T26 {"Visible?"=FALSE} ("Set Run-Time Menu Visibility Argument"), "Visible?"=w217) -> (w218:T26)
            n100 = call-poly <vilib>:"Delacor_lib_QMH_Enqueue Message (poly).vi"("Message Data"=w218, "Message"="Set Run-Time Menu Visibility", "Message Queue in"=w221) -> ("error out"=w222:errorcluster)  [unwired: 7 in, 1 out]
          }
          event User Event {
            # "Another Module called the \"Set Window Closeable State\" API Method."
            n101 = event-data() -> ("Closeable?"=w223:bool)  [unwired: 1 in]
            n102 = Bundle(cluster=T27 {"Closeable?"=FALSE} ("Set Window Closeable State Argument"), "Closeable?"=w223) -> (w224:T27)
            n103 = call-poly <vilib>:"Delacor_lib_QMH_Enqueue Message (poly).vi"("Message Data"=w224, "Message"="Set Window Closeable State", "Message Queue in"=w227) -> ("error out"=w228:errorcluster)  [unwired: 7 in, 1 out]
          }
          event User Event {
            # "Another Module called the \"Shutdown Application\" API Method."
            n104 = event-data() -> ("User Confirm?"=w229:bool)  [unwired: 1 in]
            n105 = Bundle(cluster=T9 {"User Confirm?"=FALSE} ("Shutdown Application Argument"), "User Confirm?"=w229) -> (w230:T9)
            n106 = call-poly <vilib>:"Delacor_lib_QMH_Enqueue Message (poly).vi"("Message Data"=w230, "Message"="Shutdown Application", "Message Queue in"=w233) -> ("error out"=w234:errorcluster)  [unwired: 7 in, 1 out]
          }
          event User Event {
            # "Another Module called the \"Remove Module from Run-Time Menu\" API Method."
            n107 = event-data() -> ("Module DQMH Path"=w235:path)  [unwired: 1 in]
            n108 = Bundle(cluster=T13 {"Module DQMH Path"=path ""} ("Remove Module from Run-Time Menu Argument"), "Module DQMH Path"=w235) -> (w236:T13)
            n109 = call-poly <vilib>:"Delacor_lib_QMH_Enqueue Message (poly).vi"("Message Data"=w236, "Message"="Remove Module from Run-Time Menu", "Message Queue in"=w239) -> ("error out"=w240:errorcluster)  [unwired: 7 in, 1 out]
          }
          event User Event {
            # "Another Module called the \"Broadcast Arguments\" API Method."
            n110 = event-data() -> ("CLI Arguments"=w243:string[], "Wait Notifier"=w242:refnum<notifier>, "wait for reply"=w241:bool)  [unwired: 1 in]
            n111 = Bundle(cluster=T28 {"CLI Arguments"=[], "Wait Notifier"=refnum, "wait for reply"=FALSE} ("Broadcast Arguments Argument"), "CLI Arguments"=w243, "Wait Notifier"=w242, "wait for reply"=w241) -> (w244:T28)
            n112 = call-poly <vilib>:"Delacor_lib_QMH_Enqueue Message (poly).vi"("Message Data"=w244, "Message"="Set CLI Arguments", "Message Queue in"=w247) -> ("error out"=w248:errorcluster)  [unwired: 7 in, 1 out]
          }
          event User Event {
            # "Another Module called the \"Get CLI Arguments\" API Method."
            n113 = event-data() -> ("Wait Notifier"=w251:refnum<notifier>, "wait for reply"=w250:bool)  [unwired: 1 in]
            n114 = Bundle(cluster=T29 {"Wait Notifier"=refnum, "wait for reply"=FALSE} ("Get CLI Arguments Argument"), "Wait Notifier"=w251, "wait for reply"=w250) -> (w252:T29)
            n115 = call-poly <vilib>:"Delacor_lib_QMH_Enqueue Message (poly).vi"("Message Data"=w252, "Message"="Get CLI Arguments", "Message Queue in"=w255) -> ("error out"=w249:errorcluster)  [unwired: 7 in, 1 out]
          }
          event User Event {
            n116 = event-data() -> ("User Name"=w261:string, "User Level"=w260:string)  [unwired: 1 in]
            n117 = Bundle(cluster=T30 {"User Name"="", "User Level"=""} ("External Login Argument"), "User Name"=w261, "User Level"=w260) -> (w257:T30)
            n118 = call-poly <vilib>:"Delacor_lib_QMH_Enqueue Message (poly).vi"("Message Data"=w257, "Message"="External Login", "Message Queue in"=w259) -> ("error out"=w258:errorcluster)  [unwired: 7 in, 1 out]
          }
          event User Event {
            n119 = event-data() -> ("Wait Notifier"=w268:refnum<notifier>, "wait for reply"=w267:bool)  [unwired: 1 in]
            n120 = Bundle(cluster=T31 {"Wait Notifier"=refnum, "wait for reply"=FALSE} ("Get User Level Argument"), "Wait Notifier"=w268, "wait for reply"=w267) -> (w264:T31)
            n121 = call-poly <vilib>:"Delacor_lib_QMH_Enqueue Message (poly).vi"("Message Data"=w264, "Message"="Get User Level", "Message Queue in"=w266) -> ("error out"=w265:errorcluster)  [unwired: 7 in, 1 out]
          }
        }
        n122 = call-dynamic "Delacor_lib_QMH_Error Handler - Event Handling Loop.vi"("error in"=w39, "Message Queue in"=w34) -> ("dup error in"=w38:errorcluster)  [unwired: 8 in, 1 out]
      }
      n123 = while {
        tunnel: w25 -> [w272]
        shift-right: [w276] -> _
        shift-left: T2 {"hse-config"=refnum, "Module Paths"=[], "Default Title"="", "Layout"={"Layout-VI Ref"=refnum, "SP_Content Ref"=refnum, "Subpanel VI Ref"=refnum, "STR_Headline"=refnum, "SubPanels"={}}, "CLI Arguments"=[], "Login Argument"={"User Name"="", "User Level"=""}} ("Data Cluster") -> [w277]
        tunnel: w29 -> [w280]
        tunnel: [w278] -> w31
        tunnel: w24 -> [w270]
        stop <- w275 stop-if-true
        # "Message Handling Loop"
        n124 = call-dynamic "Delacor_lib_QMH_Dequeue Message.vi"("error in"=w280, "Message Queue in"=w272) -> ("error out"=w279:errorcluster, "Message Data"=w273:variant, "Message"=w274:string, "Message Queue out"=w271:refnum<class "Delacor_lib_QMH_Message Queue.lvclass">)  [unwired: 6 in]
        n125 = case "DQMH_MESSAGE_CASES" shown="\"Set Modules\"" w274 {
          selector: w274 -> [_ _ _ _ _ _ _ _ _ _ _ _ _ _ _ _ _ _ _ _ _ _ _ _ _ _ _ _ _ _ _ _ _ _ _ _ _ _ w758]
          tunnel: w271 -> [_ _ _ w335 _ _ _ _ _ _ _ _ _ _ _ _ _ _ _ _ _ w552 _ _ _ _ _ _ _ _ _ _ _ _ w675 _ w722 w742 _]
          tunnel: w279 -> [w300 w306 w324 w341 w357 w370 w383 w410 w417 w428 w453 w458 w466 w478 w484 w493 w502 w512 w521 w523 w532 w558 w569 w576 w578 w586 w638 w650 w654 w657 w660 w663 w669 w671 w683 w706 w725 w756 w760]
          tunnel: [w297 w306 w322 w337 w356 w373 w385 w405 w417 w426 w452 w456 w465 w471 w487 w493 w500 w510 w519 w523 w530 w543 w568 w574 w578 w584 w625 w649 w654 w656 w659 w662 w668 w671 w679 w705 w724 w751 w761] -> w281
          tunnel: w277 -> [w296 w305 w320 w329 w346 w367 w377 w402 w416 w423 w451 w455 w464 w477 w486 w492 w499 w505 w518 w522 w526 w550 w566 w573 w577 w583 w637 w641 w653 w655 w658 w661 w667 w670 w677 w703 w723 w741 w759]
          tunnel: [w295 w305 w319 w328 w347 w367 w376 w402 w416 w423 w451 w455 w464 w477 w486 w492 w499 w505 w518 w522 w526 w551 w566 w573 w577 w583 w632 w641 w653 w655 w658 w661 w667 w670 w677 w703 w723 w741 w759] -> w276
          tunnel: [_ _ _ _ _ _ _ _ _ _ _ _ _ _ _ _ _ _ _ _ _ _ _ _ _ _ _ _ _ _ _ _ _ _ _ _ _ w749 _] -> w275
          tunnel: w273 -> [_ _ _ _ w354 w364 w382 w409 _ w425 w450 _ w463 w476 _ _ w498 w509 w517 _ w529 w555 w565 w572 _ _ w636 w648 _ _ _ _ _ _ w676 w698 _ w748 _]
          tunnel: w270 -> [w288 _ _ _ _ _ _ _ _ _ _ _ _ _ _ _ _ _ _ _ _ _ _ _ _ _ _ _ _ _ _ _ _ _ w674 _ _ w743 _]
          frame "Initialize" {
            w293 = path[] []  # Module Paths
            # "Initialize - Any operation that needs to be done before the module can receive messages. Synchronize Caller Events.vi will inform Start Module.vi that the module has launched and is ready to receive messages. Module Did Init.vi will broadcast that the module initialized."
            n126 = call "Synchronize Caller Events.vi"("error in (no error)"=w300, "Singleton Module Admin in"=w288) -> ("error out"=w299:errorcluster, "Singleton Module Admin out"=w287:refnum<class "Delacor_lib_QMH_Module Admin.lvclass">)  [unwired: 8 in]
            n127 = property on="Property Node" class="Module Admin"(reference=w287, error in=w299) -> (error out=w304:errorcluster, "Accessors:External Launch"=w286:bool)  [unwired: 1 out]
            n128 = call "Module Name--constant.vi"() -> ("Module Name"=w282:string)  [unwired: 11 in]
            n129 = Select(t=T32."Hidden" ("State"), s=w286, f=T32."Standard" ("State")) -> (s? t:f=w285:T32)
            n130 = property on="Property Node" class="VI"(error in=w304, "Front Panel.Title"=w282) -> (reference out=w292:refnum<vi>, error out=w303:errorcluster)  [unwired: 1 in]
            n131 = invoke on="Invoke Node" class="VI" method="FP.Open"(reference=w292, error in=w303, "State"=w285) -> (reference out=w291:refnum<vi>, error out=w302:errorcluster)  [unwired: 2 in, 3 out]
            n132 = invoke on="Invoke Node" class="VI" method="FP.Center"(reference=w291, error in=w302) -> (error out=w301:errorcluster)  [unwired: 1 in, 2 out]
            n133 = call "Module Did Init.vi"("error in (no error)"=w301, "Initialized?"=TRUE, "Origin"=w282) -> ("error out"=w298:errorcluster)  [unwired: 8 in]
            n134 = Bundle By Name(cluster=w296, "Module Paths"=w293) -> (w295:T2)
            n135 = Format Into String(format string="Module %s initialised", w282) -> (resulting string=w283:string)  [unwired: 2 in, 1 out]
            n136 = call <vilib>:"INFO.vi"("Message"=w283, "error in"=w298) -> ("error out"=w297:errorcluster)  [unwired: 9 in]
          }
          frame "---Setup---" {
            # "Separator -- The following cases handle messages specific to this Module."
          }
          frame "Configure" {
            # "#HSE specific request: Triggers the auto-configuration of the module."
            n137 = call "hse-application_GetApplicationInfos.vi"("error in"=w324) -> ("error out"=w323:errorcluster, "Application Unit-ID"=w315:string, "Application Title"=w314:string)  [unwired: 7 in, 1 out]
            n138 = call "hse-application_GetVersionInfos.vi"("error in"=w323) -> ("error out"=w310:errorcluster, "Application Version"=→"Version":string)  [unwired: 5 in, 4 out]
            n139 = Format Into String(format string="%s (Unit %s)", w314, w315) -> (resulting string=w317:string)  [unwired: 2 in, 1 out]
            n140 = call "Module Name--constant.vi"() -> ("Module Name"=w308:string)  [unwired: 11 in]
            n141 = property on="Property Node" class="VI"("Front Panel.Title"=w317) -> ()  [unwired: 2 in, 2 out]
            n142 = call "Create Module Config.vi"("error in"=w310, "DQMH Module Name"=w308) -> ("error out"=w309:errorcluster, "config-ini out"=w307:refnum<class "config-ini.lvclass">)  [unwired: 8 in]
            n143 = control-ref of="SP_Main"() -> (w312:refnum<vi>)
            n144 = call "Load Layout.vi"("SP_Main"=w312, "error in (no error)"=w309, "hse-config"=w307) -> ("error out"=w321:errorcluster, "Layout out"=w311:T3)  [unwired: 7 in]
            n145 = Bundle By Name(cluster=w320, "Default Title"=w314, "hse-config"=w307, "Layout"=w311) -> (w319:T2)
            n146 = call <vilib>:"INFO.vi"("Message"="Module UI Manager configured.", "error in"=w321) -> ("error out"=w322:errorcluster)  [unwired: 9 in]
          }
          frame "Prepare" {
            # "#HSE specific request: Prepares the module for displaying its front panel.\nThis is based on information read from the Panels section of the configuration file."
            n147 = call-poly <vilib>:"Delacor_lib_QMH_Enqueue Message (poly).vi"("error in"=w341, "Message"="Resize", "Message Queue in"=w335) -> ("error out"=w340:errorcluster)  [unwired: 7 in, 1 out]
            n148 = Unbundle By Name(w329) -> ("Layout.SubPanels"=w327:T4, "hse-config"=w332:refnum<class "config-base.lvclass">)
            n149 = local write "Status Bar"("" ("Status Bar")) -> ()
            n150 = call "Layout - Read Panel Infos from Config.vi"("error in (no error)"=w340) -> ("error out"=w330:errorcluster, "Modules to load"=w331:string[], "Subpanel Labels"=w326:string[])  [unwired: 8 in]
            n151 = call "Layout - Load Modules into Subpanels.vi"("SubPanels - in"=w327, "error in (no error)"=w330, "Module Names"=w331, "SubPanel Names"=w326) -> ("error out"=w339:errorcluster, "SubPanels --out"=w325:T4)  [unwired: 6 in]
            n152 = Bundle By Name(cluster=w329, "Layout.SubPanels"=w325) -> (w328:T2)
            n153 = control-ref of="This VI"() -> (w333:refnum<vi>)
            n154 = call "Prepare - Load and Apply Window Settings.vi"("This VI"=w333, "error in (no error)"=w339, "hse-config"=w332) -> ("error out"=w338:errorcluster)  [unwired: 8 in]
            n155 = call "Prepare - Create Error if unable to load Subpanel.vi"("error in (no error)"=w338) -> ("error out"=w337:errorcluster)  [unwired: 10 in]
          }
          frame "Set Modules" {
            # "Lets UI know which modules are loaded so it can register for broadcast events. Can be called repeatedly to add to modules already registered for."
            n156 = Variant To Data(error in=w357, type=T18 {"Module Paths"=[path "Modules/Dummie"], "Wait Notifier"=refnum, "wait for reply"=FALSE} ("Set Modules Argument"), Variant=w354) -> (data=w352:T18, error out=w356:errorcluster)
            n157 = Unbundle By Name(w346) -> ("Module Paths"=w344:path[])
            n158 = Unbundle By Name(w352) -> ("Module Paths"=w342:path[], "Wait Notifier"=w351:refnum<notifier>, "wait for reply"=w350:bool)
            n159 = control-ref of="This Application"() -> (w343:refnum<vi>)
            n160 = call "Register Modules in UI Manager--helper.vi"("Application in"=w343, "error in (no error)"=w356, "New Modules"=w342, "Modules IN"=w344) -> ("error out"=w355:errorcluster, "Modules OUT"=w345:path[])  [unwired: 6 in]
            n161 = Bundle By Name(cluster=w346, "Module Paths"=w345) -> (w347:T2)
            n162 = Bundle By Name(cluster=T33 {"error"={"status"=FALSE, "code"=0, "source"=""}} ("Set Modules (Reply Payload)"), "error"=w355) -> (w349:T33)
            n163 = case shown="True" w350 {
              tunnel: w351 -> [_ w359]
              tunnel: w349 -> [_ w358]
              frame False {
              }
              frame True {
                n164 = Send Notification(notification=w358, notifier=w359) -> ()  [unwired: 1 in, 2 out]
              }
            }
          }
          frame "Evaluate Default Menu Selection" {
            # "forward every unhandled menu selection to project specifiv vi"
            n165 = Variant To Data(error in=w370, type=cluster{"ItemTag":string, "ItemPath":string} {"ItemTag"="", "ItemPath"=""} ("output cluster"), Variant=w364) -> (data=w362:cluster{"ItemTag":string, "ItemPath":string}, error out=w368:errorcluster)
            n166 = Unbundle(w362) -> ("ItemTag"=w360:string, "ItemPath"=w361:string)
            n167 = vi-ref "Project.lvlib:PROJECT_Evaluate Default Menu Selection.vi"() -> (w365:refnum<vi>)
            n168 = call-by-ref "?"(reference=w365, "error in"=w368, "ItemPath"=w361, "ItemTag"=w360) -> (reference out=w366:refnum<vi>, error out=w372:errorcluster, 0:"error out"=w369:errorcluster)  [unwired: 9 in]
            n169 = Close Reference(reference=w366, error in (no error)=w372) -> (error out=w371:errorcluster)
            n170 = Merge Errors(w369, w371) -> (w373:errorcluster)
          }
          frame "Set CLI Arguments" {
            # "save the CLI Arguments on the SR"
            n171 = Variant To Data(error in=w383, type=T28 {"CLI Arguments"=[], "Wait Notifier"=refnum, "wait for reply"=FALSE} ("Broadcast Arguments Argument"), Variant=w382) -> (data=w380:T28, error out=w384:errorcluster)
            n172 = Unbundle By Name(w380) -> ("CLI Arguments"=w379:string[], "Wait Notifier"=w375:refnum<notifier>, "wait for reply"=w374:bool)
            n173 = Array Size(array=w379) -> (size(s)=w378:i32)
            n174 = Bundle By Name(cluster=w377, "CLI Arguments"=w379) -> (w376:T2)
            n175 = case "array size >= 2" shown="2.." w378 {
              tunnel: w384 -> [w390 w400]
              tunnel: [w390 w399] -> w385
              tunnel: w379 -> [_ w391]
              frame Default {
                # "no - only application name, nothing of interest"
              }
              frame 2.. {
                # "convert array to string"
                # "remove eol"
                # "yes - debug arguments"
                n176 = call <vilib>:"Space Constant.vi"() -> ("String"=w393:string)
                n177 = Array To Spreadsheet String(delimiter (Tab)=w393, array=w391, 3:"\"%s\"" ("format string")) -> (spreadsheet string=w396:string)
                n178 = Search and Replace String(input string=w396, search string="\r\n") -> (result string=w395:string)  [unwired: 6 in, 3 out]
                n179 = Format Into String(format string="set CLI Arguments: %s" ("Message"), w395) -> (resulting string=w392:string)  [unwired: 2 in, 1 out]
                n180 = call <vilib>:"DEBUG.vi"("Message"=w392, "error in"=w400) -> ("error out"=w399:errorcluster)  [unwired: 9 in]
              }
            }
            n181 = case shown="True" w374 {
              tunnel: w375 -> [_ w387]
              tunnel: w385 -> [_ w386]
              frame False {
              }
              frame True {
                n182 = Bundle By Name(cluster=T34 {"error"={"status"=FALSE, "code"=0, "source"=""}} ("Set CLI Arguments (Reply Payload)"), "error"=w386) -> (w388:T34)
                n183 = Send Notification(notification=w388, notifier=w387) -> ()  [unwired: 1 in, 2 out]
              }
            }
          }
          frame "Get CLI Arguments" {
            # "requests the UI Manager to provide the CLI Arguments"
            n184 = Variant To Data(error in=w410, type=T29 {"Wait Notifier"=refnum, "wait for reply"=FALSE} ("Get CLI Arguments Argument"), Variant=w409) -> (data=w407:T29, error out=w403:errorcluster)
            n185 = Unbundle By Name(w407) -> ("wait for reply"=w404:bool, "Wait Notifier"=w406:refnum<notifier>)
            n186 = Unbundle By Name(w402) -> ("CLI Arguments"=w401:string[])
            n187 = case shown="True" w404 {
              tunnel: w406 -> [_ w415]
              tunnel: w403 -> [_ w412]
              tunnel: w401 -> [_ w411]
              frame False {
              }
              frame True {
                n188 = Bundle By Name(cluster=T35 {"CLI Arguments"=[], "error"={"status"=FALSE, "code"=0, "source"=""}} ("Get CLI Arguments (Reply Payload)"), "CLI Arguments"=w411, "error"=w412) -> (w413:T35)
                n189 = Send Notification(notification=w413, notifier=w415) -> ()  [unwired: 1 in, 2 out]
              }
            }
            n190 = Merge Errors(w403) -> (w405:errorcluster)
          }
          frame "--- UI Presentation States ---" {
            # "Separator -- The following cases handle messages specific to this Module."
          }
          frame "Update Title" {
            # "Updates the string control on the layout VI via its reference"
            n191 = Unbundle By Name(w423) -> ("hse-config"=w418:refnum<class "config-base.lvclass">, "Layout.STR_Headline"=w420:refnum<vi>, "Default Title"=w422:string)
            n192 = Variant To Data(error in=w428, type="", Variant=w425) -> (data=w421:string, error out=w427:errorcluster)
            n193 = Not A Number/Path/Refnum?(number/path/refnum=w420) -> (NaN/Path/Refnum?=w419:bool)
            n194 = case "Is the reference to the STR_Headline empty?" shown="False" w419 {
              tunnel: w427 -> [w445 w446]
              tunnel: w422 -> [w442 _]
              tunnel: w421 -> [w441 _]
              tunnel: [w443 w446] -> w426
              tunnel: w420 -> [w439 _]
              tunnel: w418 -> [w438 _]
              frame False {
                # "Not empty (valid); Update value"
                n195 = call-dynamic "Read String.vi"("Section"="global", "error in"=w445, "Key"="title_fstr", "config-base in"=w438) -> ("error out"=w435:errorcluster, "Value"=w431:string)  [unwired: 5 in, 1 out]
                n196 = call <vilib>:"Clear Errors.vi"("error in (no error)"=w435, "specific error code to clear (0: all)"=500053) -> ("error out"=w434:errorcluster)  [unwired: 4 in, 1 out]
                n197 = Empty String/Path?(string/path=w431) -> (empty?=w432:bool)
                n198 = Select(t="%s | %s" ("Section"), s=w432, f=w431) -> (s? t:f=w430:string)
                n199 = Format Into String(format string=w430, error in=w434, w442, w441) -> (resulting string=w440:string, error out=w444:errorcluster)  [unwired: 1 in]
                n200 = property on="Property Node" class="Str"(reference=w439, error in=w444, "Value"=w440) -> (error out=w443:errorcluster)  [unwired: 1 out]
              }
              frame True {
                # "Yes: Do nothing"
              }
            }
          }
          frame "Update Status Bar" {
            # "Prints a message to the status bar"
            n201 = Variant To Data(error in=w453, type=T22 {"Status Message"=""} ("Update Status Bar Argument"), Variant=w450) -> (data=w448:T22, error out=w452:errorcluster)
            n202 = Unbundle By Name(w448) -> ("Status Message"=→"Status Bar":string)
          }
          frame "Resize" {
            # "If panel is resized, redistribute columns"
            n203 = Unbundle By Name(w455) -> ("Layout.SP_Content Ref"=w454:refnum<vi>)
            n204 = invoke on="Invoke Node" class="SubPnl" method="FitControlToPane"(reference=w454, error in=w458) -> (error out=w457:errorcluster)  [unwired: 1 in, 2 out]
            n205 = invoke on="SP_Main" class="SubPnl" method="FitControlToPane"(error in=w457) -> (error out=w456:errorcluster)  [unwired: 2 in, 2 out]
          }
          frame "Set Run-Time Menu Visibility" {
            # "Sets the Visibility of the Run-Time Menu. Setting <b>Visible?</b> to true shows the menu, while setting it to false hides it."
            n206 = Variant To Data(error in=w466, type=T26 {"Visible?"=FALSE} ("Set Run-Time Menu Visibility Argument"), Variant=w463) -> (data=w461:T26, error out=w467:errorcluster)
            n207 = Unbundle By Name(w461) -> ("Visible?"=w459:bool)
            n208 = control-ref of="This VI"() -> (w460:refnum<vi>)
            n209 = property on="Property Node" class="VI"(reference=w460, error in=w467, "Front Panel.ShowMenuBar"=w459) -> (error out=w465:errorcluster)  [unwired: 1 out]
          }
          frame "Set Window Closeable State" {
            # "Disable the \"Exit\" menu entry."
            # "Disable the \"X\"."
            # "Sets the closeable state of the window. Setting <b>Closeable?</b> to true enables the close button in the title bar, while setting it to false disables it."
            n210 = Variant To Data(error in=w478, type=T27 {"Closeable?"=FALSE} ("Set Window Closeable State Argument"), Variant=w476) -> (data=w474:T27, error out=w479:errorcluster)
            n211 = Unbundle By Name(w474) -> ("Closeable?"=w468:bool)
            n212 = control-ref of="This VI"() -> (w473:refnum<vi>)
            n213 = property on="Property Node" class="VI"(reference=w473, error in=w479, "Front Panel.Closeable"=w468) -> (error out=w472:errorcluster)  [unwired: 1 out]
            n214 = Current VI's Menubar() -> (w470:refnum<k9>)
            n215 = Set Menu Item Info(7:"Exit" ("item tag"), 8:w472, 9:w468, 11:w470) -> (0:w471:errorcluster)  [unwired: 3 in, 1 out]
          }
          frame "Fade-in" {
            n216 = Unbundle By Name(w486) -> ("hse-config"=w483:refnum<class "config-base.lvclass">)
            n217 = call-dynamic "Read Boolean.vi"("Section"="global", "error in"=w484, "Key"="smooth_fade_in", "config-base in"=w483) -> ("error out"=w485:errorcluster, "Value"=w480:bool)  [unwired: 5 in, 1 out]
            n218 = case shown="True" w480 {
              tunnel: [w488 w490] -> w487
              tunnel: w485 -> [w488 w489]
              frame False {
              }
              frame True {
                n219 = control-ref of="This VI"() -> (w491:refnum<vi>)
                n220 = call "Fade-in UI.vi"("error in"=w489, "This VI"=w491) -> ("error out"=w490:errorcluster)  [unwired: 9 in]
              }
            }
          }
          frame "--- Run-Time Menu ---" {
            # "Separator -- The following cases handle messages specific to this Module."
          }
          frame "Set Run-Time Menu" {
            # "Loads the Run-Time Menu set in <b>Run-Time Menu Path</b>"
            n221 = Variant To Data(error in=w502, type=T19 {"Run-Time Menu Path"=path ""} ("Set Run-Time Menu Argument"), Variant=w498) -> (data=w496:T19, error out=w501:errorcluster)
            n222 = Unbundle By Name(w496) -> ("Run-Time Menu Path"=w494:path)
            n223 = control-ref of="This VI"() -> (w495:refnum<vi>)
            n224 = property on="Property Node" class="VI"(reference=w495, error in=w501, "RT Menu Path"=w494) -> (error out=w500:errorcluster)  [unwired: 1 out]
          }
          frame "Add Module to Run-Time Menu" {
            # "Add module options (show in subpanel, open window, show BD) to the Run-Time Menu"
            n225 = Variant To Data(error in=w512, type=T11 {"Module DQMH Path"=path "", "Module Descriptor"=""} ("Add Module to Run-Time Menu Argument"), Variant=w509) -> (data=w507:T11, error out=w511:errorcluster)
            n226 = Unbundle By Name(w507) -> ("Module DQMH Path"=w504:path, "Module Descriptor"=w503:string)
            n227 = Current VI's Menubar() -> (w506:refnum<k9>)
            n228 = call "Run-Time Menu - Create entries for module--helper.vi"("Menu in"=w506, "error in"=w511, "Module Descriptor"=w503, "Module DQMH Path"=w504) -> ("error out"=w510:errorcluster)  [unwired: 7 in]
          }
          frame "Remove Module from Run-Time Menu" {
            # "Removes all run-time menu entries for the given module"
            n229 = Variant To Data(error in=w521, type=T13 {"Module DQMH Path"=path ""} ("Remove Module from Run-Time Menu Argument"), Variant=w517) -> (data=w515:T13, error out=w520:errorcluster)
            n230 = Unbundle By Name(w515) -> ("Module DQMH Path"=w514:path)
            n231 = Current VI's Menubar() -> (w513:refnum<k9>)
            n232 = call "Run-Time Menu - Remove Module Entry--helper.vi"("Menu in"=w513, "error in"=w520, "Module DQMH Path"=w514) -> ("error out"=w519:errorcluster)  [unwired: 8 in]
          }
          frame "--- Module Display ---" {
            # "Separator -- The following cases handle messages specific to this Module."
          }
          frame "Display another Module UI" {
            # "Requests another module to display its UI in the given <b>Display Scenario</b>: The \"Stand-Alone\" scenario asks the module to open its front panel as a new windows. The \"Managed\" scenario asks the module to broadcast a request for display which the UI Manager then processes, showing the module in its subpanel."
            n233 = Variant To Data(error in=w532, type=T24 {"Module DQMH Path"=path "", "Display Scenario"=enum."Stand-Alone"} ("Display Module UI Argument"), Variant=w529) -> (data=w527:T24, error out=w531:errorcluster)
            n234 = Unbundle By Name(w527) -> ("Module DQMH Path"=w525:path, "Display Scenario"=w524:T25)
            n235 = call "Display Another Module VI--helper.vi"("error in (no error)"=w531, "Display Scenario"=w524, "Module DQMH Path"=w525) -> ("error out"=w530:errorcluster)  [unwired: 7 in, 1 out]
          }
          frame "Load Module into Subpanel" {
            # "Use custom title?"
            # "Displays a DQMH module in the subpanel"
            n236 = Variant To Data(error in=w558, type=T15 {"Module Path"=path "", "Module Name"="", "Title"="", "VI Reference"=refnum, "Target SP Name"=""} ("Load Module Into Subpanel Argument"), Variant=w555) -> (data=w554:T15, error out=w557:errorcluster)
            n237 = Unbundle By Name(w554) -> ("Target SP Name"=w534:string, "VI Reference"=w533:refnum<vi>, "Title"=w537:string, "Module Path"=w540:path)
            n238 = Strip Path(path=w540) -> (name=w547:string)  [unwired: 1 out]
            n239 = Not Equal?(x=w537, y="<not specified>" ("x")) -> (x != y?=w538:bool)
            n240 = Unbundle By Name(w550) -> ("Layout.SubPanels"=w536:T4)
            n241 = Select(t=w537, s=w538, f=w547) -> (s? t:f=w546:string)
            n242 = call "Layout - Module Into Subpanel.vi"("SubPanels in"=w536, "error in"=w557, "VI in"=w533, "Target SP Name"=w534) -> ("error out"=w545:errorcluster, "Removed Module"=w549:string, "SubPanels out"=w535:T4)  [unwired: 5 in]
            n243 = Bundle By Name(cluster=w550, "Layout.SubPanels"=w535) -> (w551:T2)
            n244 = Empty String/Path?(string/path=w549) -> (empty?=w548:bool)
            n245 = case "VI removed?" shown="False" w548 {
              tunnel: w549 -> [w559 _]
              frame False {
                # "YES"
                n246 = call "DQMH System Message - Removed from Subpanel.vi"("Removed Module"=w559) -> ("Payload"=w562:variant, "Identifier"=w561:string, "Source"=w560:T39)  [unwired: 8 in]
                n247 = call "System Message.vi"("Sys. Msg. Source"=w560, "Payload"=w562, "Identifier"=w561) -> ()  [unwired: 8 in, 1 out]
              }
              frame True {
                # "NO"
              }
            }
            n248 = call-poly <vilib>:"Delacor_lib_QMH_Enqueue Message (poly).vi"("error in"=w545, "Message Data"=w546, "Message"="Update Title", "Message Queue in"=w552) -> ("error out"=w544:errorcluster, "Message Queue out"=w542:refnum<class "Delacor_lib_QMH_Message Queue.lvclass">)  [unwired: 6 in]
            n249 = call-poly <vilib>:"Delacor_lib_QMH_Enqueue Message (poly).vi"("error in"=w544, "Message"="Fade-in", "Message Queue in"=w542) -> ("error out"=w543:errorcluster)  [unwired: 7 in, 1 out]
          }
          frame "Show Module Diagram" {
            w563 = path ""  # Module DQMH Path
            # "Requests a module to show its block diagram (called from run-time menu)"
            n250 = Variant To Data(error in=w569, type=w563, Variant=w565) -> (data=w564:path, error out=w567:errorcluster)
            n251 = call "Show Module Diagram--helper.vi"("error in (no error)"=w567, "Module DQMH Path"=w564) -> ("error out"=w568:errorcluster)  [unwired: 9 in]
          }
          frame "Load API Tester" {
            w570 = path ""  # Module DQMH Path
            # "Opens a reference to a module's API Tester VI and runs it asynchronously (called from run-time menu)"
            n252 = Variant To Data(error in=w576, type=w570, Variant=w572) -> (data=w571:path, error out=w575:errorcluster)
            n253 = call "Load API Tester--helper.vi"("error in (no error)"=w575, "Module DQMH Path"=w571) -> ("error out"=w574:errorcluster)  [unwired: 9 in]
          }
          frame "--- User Authentication ---" {
            # "Separator -- The following cases handle messages specific to this Module."
          }
          frame "Login" {
            w579 = "Enter Credentials"  # Title
            # "checks the credentials entered by a user against the project-specific credentials file"
            n254 = call "Dialogue_UserCredentials.vi"("error in"=w586, "Title"=w579) -> ("error out"=w585:errorcluster, "Cancelled?"=w582:bool, "Password OUT"=w580:string, "Username OUT"=w581:string)  [unwired: 6 in]
            n255 = case "Did user cancel input?" shown="False" w582 {
              tunnel: [w588 w620] -> w584
              tunnel: w585 -> [w601 w620]
              tunnel: w581 -> [w589 _]
              tunnel: w580 -> [w597 _]
              frame False {
                # "No: Check Credentials"
                n256 = vi-ref "Project.lvlib:PROJECT_UserCredentials.vi"() -> (w594:refnum<vi>)
                n257 = call-by-ref "?"(reference=w594, "error in"=w601, "Password"=w597, "Username"=w589) -> (reference out=w598:refnum<vi>, error out=w604:errorcluster, 0:"error out"=w603:errorcluster, "Userlevel"=w595:string)  [unwired: 8 in]
                n258 = Close Reference(reference=w598, error in (no error)=w604) -> (error out=w602:errorcluster)
                n259 = Merge Errors(w603, w602) -> (w599:errorcluster)
                n260 = Format Into String(format string="Logged in as \"%s\"", w589) -> (resulting string=w593:string)  [unwired: 2 in, 1 out]
                n261 = Empty String/Path?(string/path=w595) -> (empty?=w596:bool)
                n262 = Not(x=w596) -> (.not. x?=w591:bool)
                n263 = Current VI's Menubar() -> (w590:refnum<k9>)
                n264 = case "Are the credentials valid?" shown="True" w591 {
                  tunnel: [w608 w617] -> w600
                  tunnel: w595 -> [_ w610]
                  tunnel: w599 -> [w609 w619]
                  tunnel: w593 -> [_ w616]
                  tunnel: w590 -> [w606 w614]
                  tunnel: w589 -> [_ w611]
                  tunnel: ["Authentication attempt failed." w612] -> w587
                  frame False {
                    w607 = FALSE  # disable
                    # "No: Disable API Tester"
                    n265 = call "Run-Time Menu - Toggle API Tester Enabled--helper.vi"("error in (no error)"=w609, "enabled"=w607, "Menu in"=w606) -> ("error out"=w608:errorcluster)  [unwired: 8 in]
                  }
                  frame True {
                    w615 = TRUE  # enabled
                    # "Yes: Propagate login level"
                    n266 = call "Login.vi"("error in (no error)"=w619, "User Name"=w611, "User Level"=w610) -> ("error out"=w618:errorcluster)  [unwired: 8 in]
                    n267 = local write "Status Bar"(w616) -> ()
                    n268 = call "Run-Time Menu - Toggle API Tester Enabled--helper.vi"("error in (no error)"=w618, "enabled"=w615, "Menu in"=w614) -> ("error out"=w617:errorcluster)  [unwired: 8 in]
                    n269 = Format Into String(format string="User \"%s\" logged in as \"%s\".", w611, w610) -> (resulting string=w612:string)  [unwired: 2 in, 1 out]
                  }
                }
                n270 = call <vilib>:"INFO.vi"("Message"=w587, "error in"=w600) -> ("error out"=w588:errorcluster)  [unwired: 9 in]
              }
              frame True {
                # "Yes: user cancelled the process"
              }
            }
          }
          frame "External Login" {
            # "User logged in from another module"
            n271 = Variant To Data(error in=w638, type=T30 {"User Name"="", "User Level"=""} ("External Login Argument"), Variant=w636) -> (data=w634:T30, error out=w633:errorcluster)
            n272 = Unbundle By Name(w634) -> ("User Level"=w622:string, "User Name"=w621:string)
            n273 = Bundle By Name(cluster=w637, "Login Argument.User Level"=w622, "Login Argument.User Name"=w621) -> (w632:T2)
            n274 = Empty String/Path?(string/path=w622) -> (empty?=w630:bool)
            n275 = Format Into String(format string="Logged in as \"%s\"" ("Format-String"), w621) -> (resulting string=w629:string)  [unwired: 2 in, 1 out]
            n276 = Select(t="Logged out", s=w630, f=w629) -> (s? t:f=w627:string)
            n277 = call "Login.vi"("error in (no error)"=w633, "User Name"=w621, "User Level"=w622) -> ("error out"=w626:errorcluster)  [unwired: 8 in]
            n278 = local write "Status Bar"(w627) -> ()
            n279 = Format Into String(format string="User \"%s\" logged in as \"%s\".", w621, w622) -> (resulting string=w624:string)  [unwired: 2 in, 1 out]
            n280 = call <vilib>:"INFO.vi"("Message"=w624, "error in"=w626) -> ("error out"=w625:errorcluster)  [unwired: 9 in]
          }
          frame "Get User Level" {
            # "Returns the User credentials to the requester"
            n281 = Variant To Data(error in=w650, type=T31 {"Wait Notifier"=refnum, "wait for reply"=FALSE} ("Get User Level Argument"), Variant=w648) -> (data=w647:T31, error out=w649:errorcluster)
            n282 = Unbundle By Name(w647) -> ("Wait Notifier"=w644:refnum<notifier>, "wait for reply"=w645:bool)
            n283 = Unbundle By Name(w641) -> ("Login Argument.User Name"=w640:string, "Login Argument.User Level"=w639:string)
            n284 = Bundle By Name(cluster=T36 {"User Name"="", "User Level"="", "error"={"status"=FALSE, "code"=0, "source"=""}} ("Get User Level (Reply Payload)"), "User Name"=w640, "User Level"=w639) -> (w642:T36)
            n285 = case shown="True" w645 {
              tunnel: w644 -> [_ w652]
              tunnel: w642 -> [_ w651]
              frame False {
              }
              frame True {
                n286 = Send Notification(notification=w651, notifier=w652) -> ()  [unwired: 1 in, 2 out]
              }
            }
          }
          frame "--- Dialogs ---" {
            # "Separator -- The following cases handle messages specific to this Module."
          }
          frame "Show HSE-ABOUT" {
            # "Shows the About window of Hampel Software Engineering"
            n287 = call "Screen_ShowHseAbout.vi"("error in"=w657) -> ("error out"=w656:errorcluster)  [unwired: 10 in]
          }
          frame "Show PROJECT-ABOUT" {
            # "Shows the About window of this application"
            n288 = call "Screen_ShowProjectAbout.vi"("error in"=w660) -> ("error out"=w659:errorcluster)  [unwired: 10 in]
          }
          frame "---Debug/Demo---" {
            # "Duplicate this frame when creating new messages.  Change this comment in the duplicated frame to describe this message."
            n289 = Merge Errors(w663) -> (w662:errorcluster)
          }
          frame "Trigger System Message" {
            w664 = variant  # Payload
            w665 = "This is a demo broadcast"  # Identifier
            w666 = System_Message_Source."module"  # Source
            # "Manually triggers a System Message broadcast event.\nThis case exists only for the purpose of showcasing the ActorModule's features."
            n290 = call "System Message.vi"("Sys. Msg. Source"=w666, "error in (no error)"=w669, "Payload"=w664, "Identifier"=w665) -> ("error out"=w668:errorcluster)  [unwired: 7 in]
          }
          frame "--- Exit and Error Handling---" {
            # "Separator - The following cases handle errors and exit messages."
          }
          frame "Error" {
            # "Error - Check the error message data and respond accordingly. This message is sent by the \"Error Handler\" VIs at the end of each loop in this application."
            n291 = property on="Property Node" class="Module Admin"(reference=w674) -> ("Accessors:External Launch"=w673:bool)  [unwired: 1 in, 2 out]
            n292 = Variant To Data(error in=w683, type=errorcluster {"status"=FALSE, "code"=0, "source"=""} ("error constant"), Variant=w676) -> (data=w678:errorcluster, error out=w681:errorcluster)
            n293 = call "Error Reported.vi"("Error"=w678) -> ()  [unwired: 10 in, 1 out]
            n294 = case shown="False" w673 {
              tunnel: [w687 _] -> w680
              tunnel: w675 -> [w686 _]
              tunnel: w678 -> [_ w688]
              frame False {
                # "If the module is running standalone, then pop up an error dialog and call the \"Exit\" message."
                n295 = call-poly <vilib>:"Delacor_lib_QMH_Enqueue Message (poly).vi"("Priority Message? (F)"=TRUE, "Message"="Exit", "Message Queue in"=w686) -> ("error out"=w687:errorcluster)  [unwired: 7 in, 1 out]
              }
              frame True {
                # "this VI is the user interface manager, so it has to display errors by itself!"
                n296 = call "Dialogue_Error.vi"("error in"=w688) -> ()  [unwired: 10 in, 1 out]
              }
            }
            n297 = call <vilib>:"ERROR.vi"("Message"="DQMH Error Case", "error in"=w678) -> ()  [unwired: 9 in, 1 out]
            n298 = Merge Errors(w681, w680) -> (w679:errorcluster)
            n299 = local write "error out"(w679) -> ()
          }
          frame "Shutdown Application" {
            # "Don't show pop-up\nif config can't be read."
            # "Never show the popup\nif \"supress_popup\" is True."
            # "Tell the UI Manager to initiate the application shutdown sequence"
            n300 = Unbundle By Name(w703) -> ("hse-config"=w702:refnum<class "config-base.lvclass">)
            n301 = Variant To Data(error in=w706, type=T9 {"User Confirm?"=FALSE} ("Shutdown Application Argument"), Variant=w698) -> (data=w696:T9, error out=w699:errorcluster)
            n302 = Unbundle By Name(w696) -> ("User Confirm?"=w695:bool)
            n303 = call-dynamic "Read Boolean.vi"("Section"="global", "error in"=w699, "Key"="supress_popup", "config-base in"=w702) -> ("error out"=w691:errorcluster, "Value"=w693:bool)  [unwired: 5 in, 1 out]
            n304 = Unbundle By Name(w691) -> ("status"=w692:bool)
            n305 = call <vilib>:"ERROR.vi"("Message"="Config key \"supress_popup\" not found.", "error in"=w691) -> ("error out"=w690:errorcluster)  [unwired: 9 in]
            n306 = Compound Arithmetic op=AND(w695, invert w693, invert w692) -> (w694:bool)
            n307 = case "Confirmation required?" shown="True" w694 {
              tunnel: [w707 w708] -> w704
              frame False {
                w707 = TRUE  # shutdown unconditionally
                # "no: just shutdown"
              }
              frame True {
                # "yes: show popup"
                n308 = Two Button Dialog(message="Close and exit application?", 1:"Cancel" ("F button name (\"Cancel\")"), 2:"Exit" ("T button name (\"OK\")")) -> (T button?=w708:bool)
              }
            }
            n309 = case "User confirmed or no confirmation needed?" shown="True" w704 {
              tunnel: w690 -> [w712 w717]
              tunnel: [w712 w716] -> w705
              frame False {
                # "no: do nothing"
              }
              frame True {
                w713 = variant  # Payload
                w714 = System_Message_Source."module"  # Source
                # "yes: shutdown"
                n310 = call "System Message.vi"("Sys. Msg. Source"=w714, "error in (no error)"=w717, "Payload"=w713, "Identifier"="Shutdown Application") -> ("error out"=w716:errorcluster)  [unwired: 7 in]
              }
            }
          }
          frame "Confirm Quit" {
            # "Confirm Quit - Message that can confirm whether or not the user wants to exit the application."
            n311 = Two Button Dialog(message="Close and exit application?", 1:"Cancel" ("F button name (\"Cancel\")"), 2:"Exit" ("T button name (\"OK\")")) -> (T button?=w718:bool)
            n312 = case shown="True" w718 {
              tunnel: w725 -> [w726 w729]
              tunnel: [w726 w728] -> w724
              tunnel: w722 -> [_ w727]
              frame False {
              }
              frame True {
                n313 = disable-structure shown="Enabled" {
                  disable-tunnel: w729 -> [w734 w739]
                  disable-tunnel: [w733 w738] -> w728
                  disable-tunnel: w727 -> [w732 _]
                  frame Disabled {
                    n314 = call-poly <vilib>:"Delacor_lib_QMH_Enqueue Message (poly).vi"("Priority Message? (F)"=TRUE, "error in"=w734, "Message"="Exit", "Message Queue in"=w732) -> ("error out"=w733:errorcluster)  [unwired: 6 in, 1 out]
                  }
                  frame Enabled {
                    w735 = variant  # Payload
                    w736 = System_Message_Source."module"  # Source
                    n315 = call "System Message.vi"("Sys. Msg. Source"=w736, "error in (no error)"=w739, "Payload"=w735, "Identifier"="Shutdown Application") -> ("error out"=w738:errorcluster)  [unwired: 7 in]
                  }
                }
              }
            }
          }
          frame "Exit" {
            w749 = TRUE  # Stop the VI
            # "Close ref to module (main VI )shown in subpanel.\nIgnore if ref is not valid or module already stopped."
            # "Release the message queue reference"
            # "Exit - Exit the application."
            n316 = Variant To Data(error in=w756, type=T8 {"Origin"="", "Exit via Stop Module Req?"=FALSE, "Wait for Module to stop?"=FALSE} ("Stop Argument"), Variant=w748) -> (data=w745:T8, error out=w753:errorcluster)
            n317 = call <vilib>:"Clear Errors.vi"("error in (no error)"=w753, "specific error code to clear (0: all)"=91 ("91: not all Exit messages will have an argument")) -> ("error out"=w755:errorcluster)  [unwired: 4 in, 1 out]
            n318 = Unbundle By Name(w741) -> ("Layout.Subpanel VI Ref"=w740:refnum<vi>)
            n319 = control-ref of="This VI"() -> (w744:refnum<vi>)
            n320 = Close Reference(reference=w740) -> (error out=w750:errorcluster)  [unwired: 1 in]
            n321 = call "Handle Exit.vi"("Stop Argument"=w745, "Admin in"=w743, "VI reference"=w744) -> ("error out"=w752:errorcluster)  [unwired: 7 in, 1 out]
            n322 = call-dynamic "Delacor_lib_QMH_Release Message Queue.vi"("error in"=w755, "Message Queue"=w742) -> ("error out"=w754:errorcluster)  [unwired: 9 in]
            n323 = call <vilib>:"Clear Errors.vi"("error in (no error)"=w750) -> ()  [unwired: 5 in, 2 out]
            n324 = Merge Errors(w754, w752) -> (w751:errorcluster)
            n325 = call "Error Reported.vi"("Error"=w751) -> ()  [unwired: 10 in, 1 out]
          }
          frame Default {
            # "'Default' case only runs if there is a message that isn't defined in any of the other cases.  Output a programming error."
            n326 = call "Module Name--constant.vi"() -> ("Module Name"=w757:string)  [unwired: 11 in]
            n327 = xnode "Error Ring"("parameter 0"=w758, "parameter 1"=w757) -> ("error out"=w762:errorcluster)
            n328 = Merge Errors(w760, w762) -> (w761:errorcluster)
          }
        }
        n329 = call-dynamic "Delacor_lib_QMH_Error Handler - Message Handling Loop.vi"("error in"=w281, "Message Queue in"=w271) -> ("dup error in"=w278:errorcluster)  [unwired: 8 in, 1 out]
      }
    }
    frame Error {
      # "Synchronize Caller Events.vi will inform Start Module.vi that the module has launched and will let the code calling Start Module.vi register for broadcasts and would permit the caller receive the broadcast that an error occurred at launch time."
      n330 = call-dynamic "Delacor_lib_QMH_Release Message Queue.vi"("Message Queue"=w771) -> ()  [unwired: 10 in, 1 out]
      n331 = call "Synchronize Caller Events.vi"("Singleton Module Admin in"=w772) -> ("error out"=w777:errorcluster)  [unwired: 9 in, 1 out]
      n332 = call "Module Name--constant.vi"() -> ("Module Name"=w775:string)  [unwired: 11 in]
      n333 = Format Into String(format string="An error occurred during initialization. %s is no longer running.", w775) -> (resulting string=w773:string)  [unwired: 2 in, 1 out]
      n334 = Merge Errors(w779, w777) -> (w778:errorcluster)
      n335 = call "Error Reported.vi"("Additional Information"=w773, "Error"=w778) -> ()  [unwired: 9 in, 1 out]
    }
  }
  n336 = Merge Errors(w19, w22) -> (w18:errorcluster)
  n337 = call "Close Module.vi"("error in (no error)"=w18, "Module Admin in"=w12) -> ("error out"=w20:errorcluster, "External Launch"=w7:bool, "Module Admin out"=w8:refnum<class "Delacor_lib_QMH_Module Admin.lvclass">)  [unwired: 7 in]
  n338 = call "Module Name--constant.vi"() -> ("Module Name"=w2:string)  [unwired: 11 in]
  n339 = Unregister For Events(event registration refnum=w11, error in=w20) -> (error out=w14:errorcluster)
  n340 = case "External Launch?" shown="True" w7 {
    tunnel: w14 -> [_ w780]
    frame False {
    }
    frame True {
      n341 = case shown="No Error" w780 {
        frame No Error {
          n342 = invoke on="Invoke Node" class="VI" method="FP.Close"() -> ()  [unwired: 3 in, 3 out]
        }
        frame Error {
          n343 = invoke on="Invoke Node" class="VI" method="FP.Open"("Activate"=TRUE ("Activate?")) -> ()  [unwired: 4 in, 5 out]
        }
      }
    }
  }
  n344 = local write "Module Admin"(w8) -> ()
  n345 = Format Into String(format string="Module %s stopped", w2) -> (resulting string=w4:string)  [unwired: 2 in, 1 out]
  n346 = call <vilib>:"INFO.vi"("Message"=w4, "error in"=w14) -> ("error out"=→"error out":errorcluster)  [unwired: 9 in]
